vi "COM Port Selector.vi"(6 "Title":string, 7 "error in":errorcluster) -> (0 "error out":errorcluster, 3 "COM Port Selected":string)   [LabVIEW 2023]
doc: "COMSelect.vi detects all instruments with an ASRL instrument name on all local and remote machines, and allows manual selection of a particular serial port. The output of this function can then be passed into a VISA Open function to generate a VISA Reference"
panel:
  out "Title":string
  in  "OK Button":bool
  in  "COM Port Selection":u16(ring)
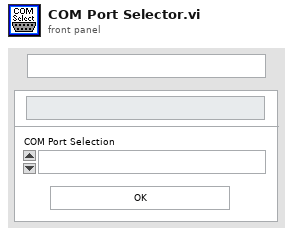
[diagram p1: front panel]
types:
  T1 = enum16{"Detect Instruments", "Open Front Panel", "Wait for User Input", "Close"}
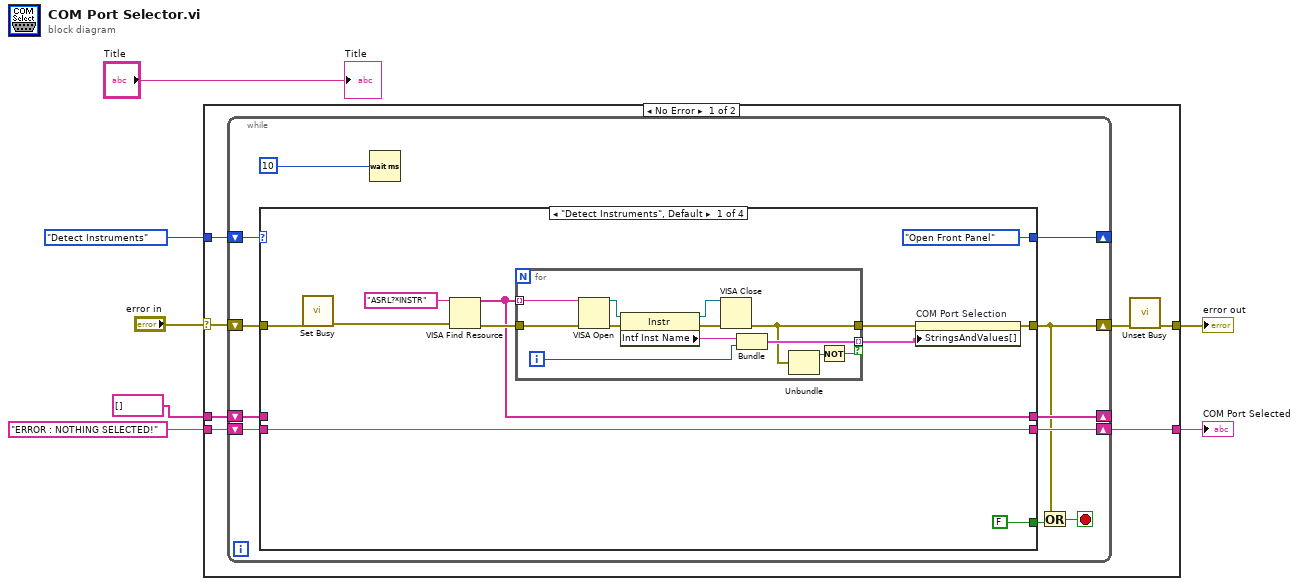
[diagram p0: block diagram]
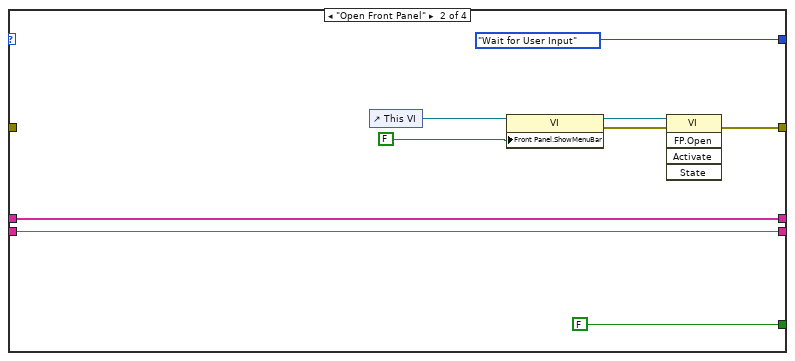
[diagram p2: hidden frame]
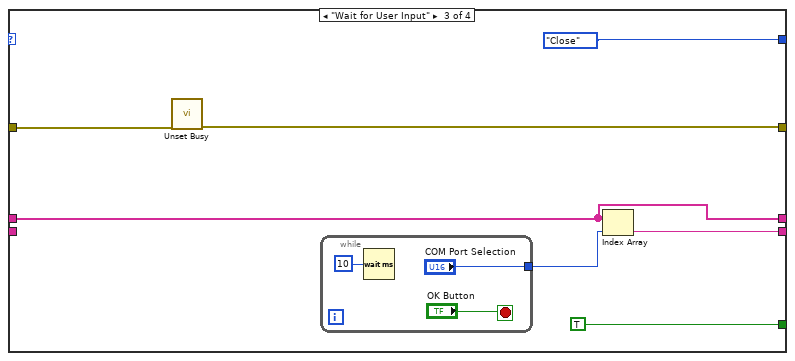
[diagram p3: hidden frame]
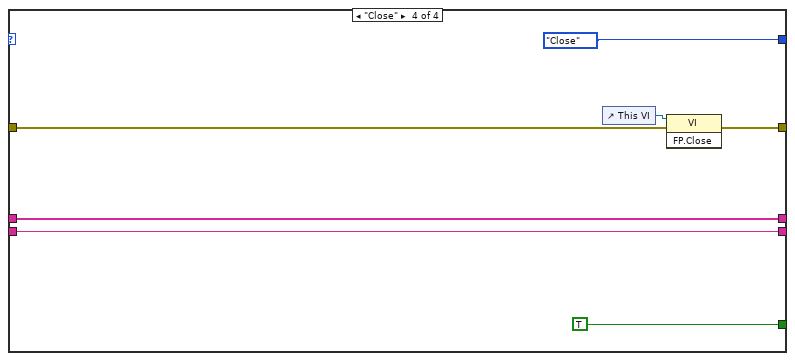
[diagram p4: hidden frame]
diagram:
  n1 = case shown="No Error" "error in" {
    selector: "error in" -> [w8 w76]
    tunnel: T1."Detect Instruments" -> [w14 _]
    tunnel: [w12 w75] -> w6
    tunnel: "ERROR : NOTHING SELECTED!" -> [w11 w75]
    tunnel: string[] [] ("find list") -> [w10 _]
    tunnel: [w9 w76] -> w2
    frame No Error {
      n2 = while {
        shift-right: [w24] -> _
        shift-left: w14 -> [w25]
        shift-right: [w15] -> w13
        shift-left: w8 -> [w23]
        shift-right: [w21] -> _
        shift-left: w10 -> [w20]
        shift-right: [w18] -> w12
        shift-left: w11 -> [w17]
        stop <- w16 stop-if-true
        n3 = case shown="\"Detect Instruments\", Default" w25 {
          tunnel: [T1."Open Front Panel" T1."Wait for User Input" T1."Close" T1."Close"] -> w24
          tunnel: w23 -> [w27 _ w59 w69]
          tunnel: [w31 w57 w58 w68] -> w15
          tunnel: [w30 w54 w60 w72] -> w21
          tunnel: w20 -> [_ w54 w60 w72]
          tunnel: [FALSE FALSE TRUE TRUE] -> w19
          tunnel: [w28 w53 w61 w71] -> w18
          tunnel: w17 -> [w28 w53 _ w71]
          frame "Detect Instruments", Default {
            n4 = call <vilib>:"Set Busy.vi"("error in (no error)"=w27) -> ("error out"=w26:errorcluster)  [unwired: 9 in, 1 out]
            n5 = VISA Find Resource(8:w26, 11:"ASRL?*INSTR" ("expression (\"?*\")")) -> (0:w35:errorcluster, 3:w30:string[])  [unwired: 2 out]
            n6 = for {
              tunnel: w30 -> [w48] mode=indexing
              tunnel: w35 -> [w46]
              tunnel: [w41] -> w36 mode=indexing if=w37
              tunnel: [w39] -> w32
              i -> [w42]
              n7 = VISA Open(error in (no error)=w46, VISA resource name=w48) -> (VISA resource name=w47:refnum<visa-resource-name>, error out=w45:errorcluster)  [unwired: 3 out]
              n8 = property class="Instr"(reference=w47, error in=w45) -> (reference out=w43:refnum<visa-resource-name>, error out=w44:errorcluster, "Intf Inst Name"=w40:string)
              n9 = VISA Close(VISA resource name=w43, error in (no error)=w44) -> (error out=w39:errorcluster)
              n10 = Bundle("Intf Inst Name"=w40, w42) -> (w41:cluster{"Intf Inst Name":string, i32})  [unwired: 1 out]
              n11 = Unbundle(w39) -> ("status"=w38:bool)  [unwired: 2 out]
              n12 = Not(x=w38) -> (.not. x?=w37:bool)
            }
            n13 = property on="COM Port Selection" class="Ring (strict)"(error in=w32, "StringsAndValues[]"=w36) -> (error out=w31:errorcluster)  [unwired: 1 in, 1 out]
          }
          frame "Open Front Panel" {
            n14 = control-ref of="This VI"() -> (w50:refnum<vi>)
            n15 = property class="VI"(reference=w50, "Front Panel.ShowMenuBar"=FALSE ("Front Panel Window:Show Menu Bar")) -> (reference out=w51:refnum<vi>, error out=w52:errorcluster)  [unwired: 1 in]
            n16 = invoke class="VI" method="FP.Open"(reference=w51, error in=w52) -> (error out=w57:errorcluster)  [unwired: 3 in, 4 out]
          }
          frame "Wait for User Input" {
            n17 = call <vilib>:"Unset Busy.vi"("error in (no error)"=w59) -> ("error out"=w58:errorcluster)  [unwired: 10 in]
            n18 = while {
              tunnel: ["COM Port Selection"] -> w64
              stop <- "OK Button" stop-if-true
              n19 = Wait (ms)(milliseconds to wait=u32 10 ("millisecond multiple")) -> ()  [unwired: 1 out]
            }
            n20 = Index Array(array=w60, index=w64) -> (element=w61:string)
          }
          frame "Close" {
            n21 = control-ref of="This VI"() -> (w70:refnum<vi>)
            n22 = invoke class="VI" method="FP.Close"(reference=w70, error in=w69) -> (error out=w68:errorcluster)  [unwired: 1 in, 2 out]
          }
        }
        n23 = Wait (ms)(milliseconds to wait=u32 10 ("millisecond multiple")) -> ()  [unwired: 1 out]
        n24 = Or(x=w15, y=w19) -> (x .or. y?=w16:bool)
      }
      n25 = call <vilib>:"Unset Busy.vi"("error in (no error)"=w13) -> ("error out"=w9:errorcluster)  [unwired: 10 in]
    }
    frame Error {
    }
  }
  "error out" <- w2
  "COM Port Selected" <- w6
  "Title" <- "Title"
